vi "Run Command.vi"(8 "error in (no error)":errorcluster, 10 "command":T1, 11 "Thread in":refnum<class "Thread.lvclass">) -> (0 "error out":errorcluster, 1 "shutdown?":bool, 3 "Thread out":refnum<class "Thread.lvclass">)   [LabVIEW 2021, in "DSF Core.lvlib" / "Thread.lvclass"]
uses:
  Thread.lvclass
  Thread Command.ctl
  Thread State.ctl
  Thread.lvclass/Thread.ctl
  <vilib>/NI/Memory Manager/Classes/Pointer/Pointer.lvclass/Pointer.ctl
  <vilib>/NI/Memory Manager/Classes/Pointer/Write.vi
  <vilib>/NI/Memory Manager/Classes/Pointer/Write U8.vi
  <vilib>/NI/Memory Manager/Classes/Pointer/Write (No Check).vi
  <vilib>/NI/Memory Manager/Classes/Pointer/Write (No Check) U8.vi
  <vilib>/NI/Memory Manager/Classes/Pointer/Check Move.vi
  <vilib>/NI/Memory Manager/Classes/Pointer/Get Address.vi
  <vilib>/NI/Memory Manager/Classes/Pointer/Check Null Pointer.vi
  <vilib>/NI/Memory Manager/Classes/Pointer/Check Count.vi
  <vilib>/NI/Memory Manager/Classes/Pointer/Check Bounds (Power of 2).vi
  <vilib>/NI/Memory Manager/Classes/Pointer/Errors.vi
  <vilib>/NI/Memory Manager/Classes/Pointer/Null Pointer.vi
  <vilib>/NI/Memory Manager/Classes/Pointer/Is Null.vi
  <vilib>/NI/Memory Manager/Classes/Pointer/Get Size.vi
  <vilib>/NI/Memory Manager/Classes/Pointer/Out of Bounds.vi
  <vilib>/NI/Memory Manager/Classes/Pointer/Check Bounds.vi
  <vilib>/NI/Memory Manager/Classes/Pointer/Create Error.vi
  <vilib>/NI/Memory Manager/VIs/Write String to Source.vi
  <vilib>/NI/Memory Manager/Classes/Pointer/Write Pointer Size to Error.vi
  <vilib>/NI/Memory Manager/VIs/Write Numeric to Source.vi
  <vilib>/NI/Memory Manager/VIs/Write Numeric Scalar to Source (Base10 U64).vi
  <vilib>/NI/Memory Manager/Classes/Pointer/Check Bounds (Pointer).vi
  <vilib>/NI/Memory Manager/Classes/Pointer/Check Bounds (Buffer).vi
  <vilib>/NI/Memory Manager/VIs/New Error Cluster.vi
  <vilib>/NI/Memory Manager/VIs/New Error Cluster (512B).vi
  <vilib>/NI/Memory Manager/VIs/Set Error Status.vi
  <vilib>/NI/Memory Manager/VIs/Set Error Code.vi
  <vilib>/NI/Memory Manager/VIs/Set Error Source.vi
  <vilib>/NI/Memory Manager/Constants/Constants.vi
  <vilib>/NI/Memory Manager/Constants/Library Name.vi
  <vilib>/NI/Memory Manager/Classes/Pointer/Pointer Error Info.vi
  <vilib>/NI/Memory Manager/Constants/Pointer Class Name.vi
  <vilib>/NI/Memory Manager/Classes/Pointer/Buffer Underflow.vi
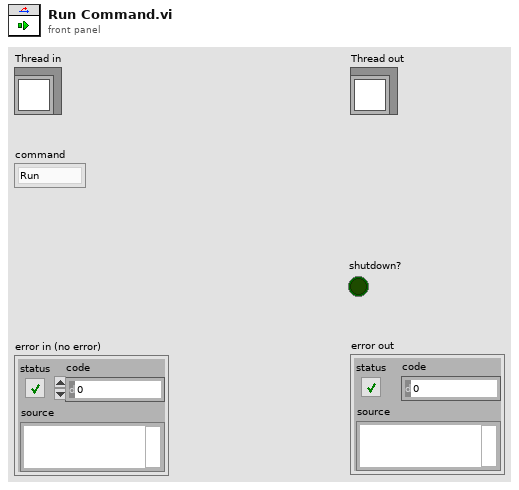
[diagram p1: front panel]
types:
  T1 = typedef "DSF Core.lvlib/Thread.lvclass/Thread Command.ctl" = enum8{"Run", "Shutdown"}
  T2 = typedef "DSF Core.lvlib/Thread.lvclass/Thread State.ctl" = enum8{"Idle", "Running", "Error", "Shut Down"}
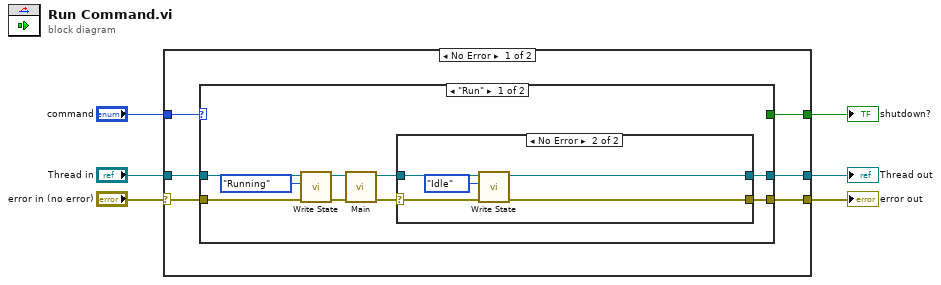
[diagram p0: block diagram]
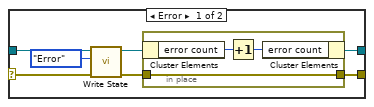
[diagram p2: hidden frame]
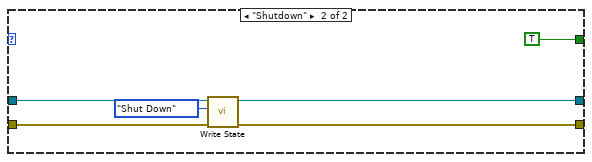
[diagram p3: hidden frame]
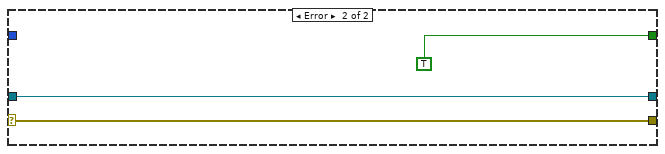
[diagram p4: hidden frame]
diagram:
  n1 = case shown="No Error" "error in (no error)" {
    selector: "error in (no error)" -> [w7 w45]
    tunnel: "command" -> [w12 _]
    tunnel: "Thread in" -> [w11 w44]
    tunnel: [w10 w44] -> w4
    tunnel: [w9 w45] -> w3
    tunnel: [w8 TRUE] -> w2
    frame No Error {
      n2 = case shown="\"Run\"" w12 {
        tunnel: w7 -> [w20 w39]
        tunnel: [w13 w37] -> w9
        tunnel: [w14 w38] -> w10
        tunnel: w11 -> [w21 w40]
        tunnel: [_ TRUE] -> w8
        frame "Run" {
          n3 = call "Write State.vi"("error in (no error)"=w20, "state"=Thread_State."Running", "Thread in"=w21) -> ("error out"=w18:errorcluster, "Thread out"=w19:refnum<class "Thread.lvclass">)  [unwired: 7 in]
          n4 = call-dynamic "Main.vi"("error in (no error)"=w18, "Thread in"=w19) -> ("error out"=w16:errorcluster, "Thread out"=w15:refnum<class "Thread.lvclass">)  [unwired: 8 in]
          n5 = case shown="No Error" w16 {
            selector: w16 -> [w26 w34]
            tunnel: w15 -> [w27 w35]
            tunnel: [w24 w33] -> w14
            tunnel: [w22 w32] -> w13
            frame Error {
              n6 = call "Write State.vi"("error in (no error)"=w26, "state"=Thread_State."Error", "Thread in"=w27) -> ("error out"=w23:errorcluster, "Thread out"=w25:refnum<class "Thread.lvclass">)  [unwired: 7 in]
              n7 = in-place {
                in-place-border: w23 -> [w29]
                in-place-border: [w29] -> w22
                n8 = in-place-cluster #1(w25) -> ("error count"=w31:i32)
                n9 = Increment(x=w31) -> (x+1=w30:i32)
                n10 = in-place-cluster #1("error count"=w30) -> (w24:refnum<class "Thread.lvclass">)
              }
            }
            frame No Error {
              n11 = call "Write State.vi"("error in (no error)"=w34, "state"=Thread_State."Idle", "Thread in"=w35) -> ("error out"=w32:errorcluster, "Thread out"=w33:refnum<class "Thread.lvclass">)  [unwired: 7 in]
            }
          }
        }
        frame "Shutdown" {
          n12 = call "Write State.vi"("error in (no error)"=w39, "state"=Thread_State."Shut Down", "Thread in"=w40) -> ("error out"=w37:errorcluster, "Thread out"=w38:refnum<class "Thread.lvclass">)  [unwired: 7 in]
        }
      }
    }
    frame Error {
    }
  }
  "Thread out" <- w4
  "error out" <- w3
  "shutdown?" <- w2
